vi "GFITS_CreateImage.vi"(0 "image name":string, 1 "multiple extensions":bool, 3 "logfile":path, 5 "imagesize(bytes)":i32, 7 "retries on error":i16=20, 9 "amplifiers":u64, 11 "error in (no error)":errorcluster, 12 "datatype":i32, 13 "totkeys":i32, 14 "hdutype":i32) -> (4 "image name out":string, 6 "return value":u64, 15 "error out":errorcluster)   [LabVIEW 2016]
panel:
  in  "newimsep":string="-"
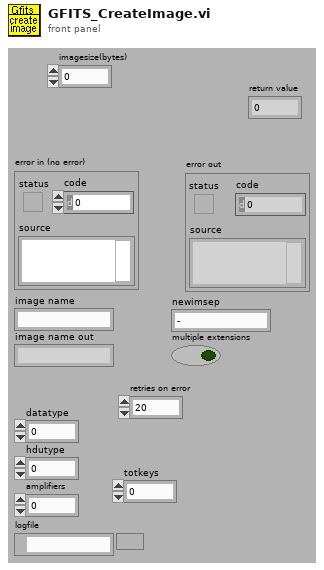
[diagram p1: front panel]
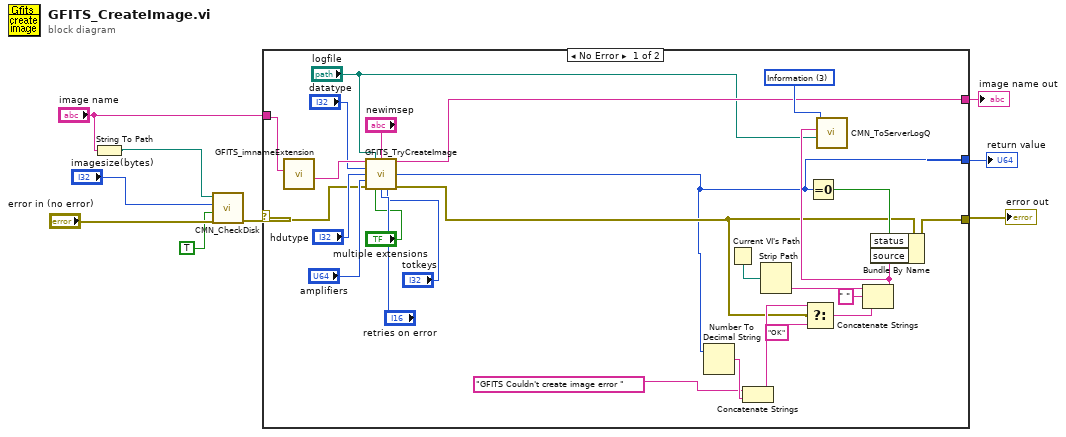
[diagram p0: block diagram]
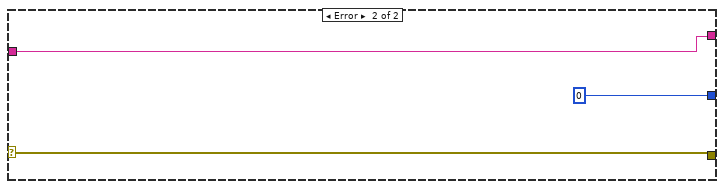
[diagram p2: hidden frame]
diagram:
  n1 = String To Path(string="image name") -> (path=w3:path)
  n2 = call "CMN_CheckDisk.vi"("error in"="error in (no error)", "Generate Error?"=TRUE, "size in"="imagesize(bytes)", "path"=w3) -> ("error out"=w5:errorcluster)  [unwired: 2 in, 5 out]
  n3 = case shown="No Error" w5 {
    selector: w5 -> [w17 w38]
    tunnel: [w13 u64 0] -> w9
    tunnel: [w33 w38] -> w8
    tunnel: [w14 w36] -> w7
    tunnel: "image name" -> [w28 w36]
    frame No Error {
      w27 = u16 3 items=["command", "imediateReply", "Callback Reply", "Information"] ("type")
      n4 = call "GFITS_imnameExtension.vi"("imname in"=w28) -> ("rootname (no extension)"=w21:string)  [unwired: 9 out]
      n5 = call "GFITS_TryCreateImage.vi"("rootname"=w21, "logfile"="logfile", "newimsep"="newimsep", "datatype"="datatype", "hdutype"="hdutype", "amplifiers"="amplifiers", "error in (no error)"=w17, "multiple extensions"="multiple extensions", "retries on error"="retries on error", "totkeys"="totkeys") -> ("imname out"=w14:string, "return value"=w13:u64, "error out"=w16:errorcluster)  [unwired: 3 out]
      n6 = Number To Decimal String(number=w13) -> (decimal integer string=w25:string)  [unwired: 1 out]
      n7 = Current VI's Path() -> (path=w34:path)
      n8 = Concatenate Strings("GFITS Couldn't create image error ", w25) -> (w23:string)
      n9 = Strip Path(path=w34) -> (name=w32:string)  [unwired: 1 out]
      n10 = Select(t=w23, s=w16, f="OK") -> (s? t:f=w29:string)
      n11 = Equal To 0?(x=w13) -> (x = 0?=w35:bool)
      n12 = Concatenate Strings(w32, " " ("string"), w29) -> (w26:string)
      n13 = call "CMN_ToServerLogQ.vi"("file"="logfile", "string"=w26, "type"=w27) -> ()  [unwired: 3 in, 5 out]
      n14 = Bundle By Name(cluster=w16, "status"=w35, "source"=w26) -> (w33:errorcluster)
    }
    frame Error {
    }
  }
  "return value" <- w9
  "error out" <- w8
  "image name out" <- w7
